vi "Simulated VeriStand Engine.Interface.Allocate.Control Pointers.vi"(8 "error in (no error)":errorcluster, 11 "Simulated VeriStand Engine Interface in":refnum<class "Simulated VeriStand Engine.Interface.lvclass">) -> (0 "error out":errorcluster, 3 "Simulated VeriStand Engine Interface out":refnum<class "Simulated VeriStand Engine.Interface.lvclass">)   [LabVIEW 2016, in "Simulated VeriStand Engine.Interface.lvclass"]
uses:
  Simulated VeriStand Engine.Interface.lvclass
  Typedefs/Simulated VeriStand Engine.Interface.Pointers.Control.ctl
  Source/Submodules/Memory/Source/Classes/Pointer/Memory.Pointer.lvclass
  Simulated VeriStand Engine.Interface.lvclass/Simulated VeriStand Engine.Interface.ctl
  Source/Submodules/Memory/Source/Classes/Pointer/Memory.Pointer.New.1B.vi
  Source/Submodules/Memory/Source/Classes/Pointer/Memory.Pointer.New.4B.vi
  Source/Submodules/Memory/Source/Classes/Pointer/Memory.Pointer.Allocate.vi
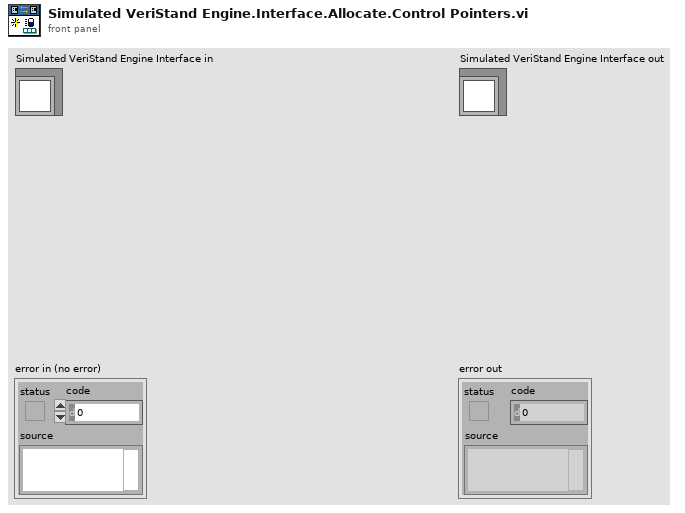
[diagram p1: front panel]
types:
  T1 = typedef "Simulated VeriStand Engine.Interface.lvclass/Simulated VeriStand Engine.Interface.Pointers.Control.ctl" = cluster{"Stop":refnum<class "Memory.Pointer.lvclass">, "Target Period (µs)":refnum<class "Memory.Pointer.lvclass">}
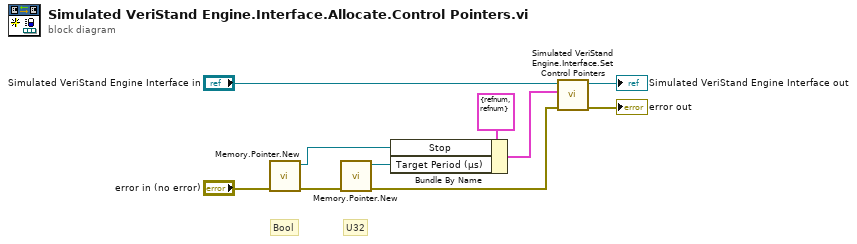
[diagram p0: block diagram]
diagram:
  # "U32"
  # "Bool"
  n1 = call-poly "Memory.Pointer.New.vi"("error in (no error)"="error in (no error)") -> ("error out"=w6:errorcluster, "pointer out"=w7:refnum<class "Memory.Pointer.lvclass">)  [unwired: 9 in]
  n2 = call-poly "Memory.Pointer.New.vi"("error in (no error)"=w6) -> ("error out"=w2:errorcluster, "pointer out"=w8:refnum<class "Memory.Pointer.lvclass">)  [unwired: 9 in]
  n3 = Bundle By Name(cluster=T1 {"Stop"=refnum, "Target Period (µs)"=refnum} ("Control Pointers"), "Stop"=w7, "Target Period (µs)"=w8) -> (w9:T1)
  n4 = call "Simulated VeriStand Engine.Interface.Set Control Pointers.vi"("error in (no error)"=w2, "Control Pointers"=w9, "Simulated VeriStand Engine Interface in"="Simulated VeriStand Engine Interface in") -> ("error out"=→"error out":errorcluster, "Simulated VeriStand Engine Interface out"=→"Simulated VeriStand Engine Interface out":refnum<class "Simulated VeriStand Engine.Interface.lvclass">)  [unwired: 7 in]
